vi "test - copy state with replace option.vi"(8 "error in (no error)":errorcluster, 11 "TestCase in":refnum<class "testcase-csmhelper.lvclass">) -> (0 "error out":errorcluster, 3 "TestCase out":refnum<class "testcase-csmhelper.lvclass">)   [LabVIEW 2017, in "testcase-csmhelper.lvclass"]
uses:
  testcase-csmhelper.lvclass
  <vilib>/addons/_JKI Toolkits/VI Tester/TestCase.llb/TestCase.lvclass
  src/user.lib/_NEVSTOP/Communicable State Machine(CSM)/Communicable State Machine.lvlib
  C:/Program Files (x86)/National Instruments/LabVIEW 2017/vi.lib/addons/_JKI Toolkits/VI Tester/TestCase.llb/TestCase.lvclass
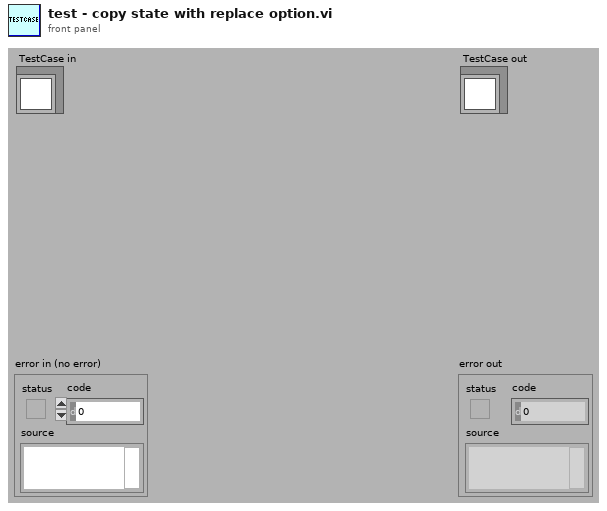
[diagram p1: front panel]
types:
  T1 = enum32{"Bad", "Idle", "Run top level", "Running"}
  T2 = cluster{"state":string, "error out":errorcluster, "Execution:State":enum32{"Bad", "Idle", "Run top level", "Running"}}[]
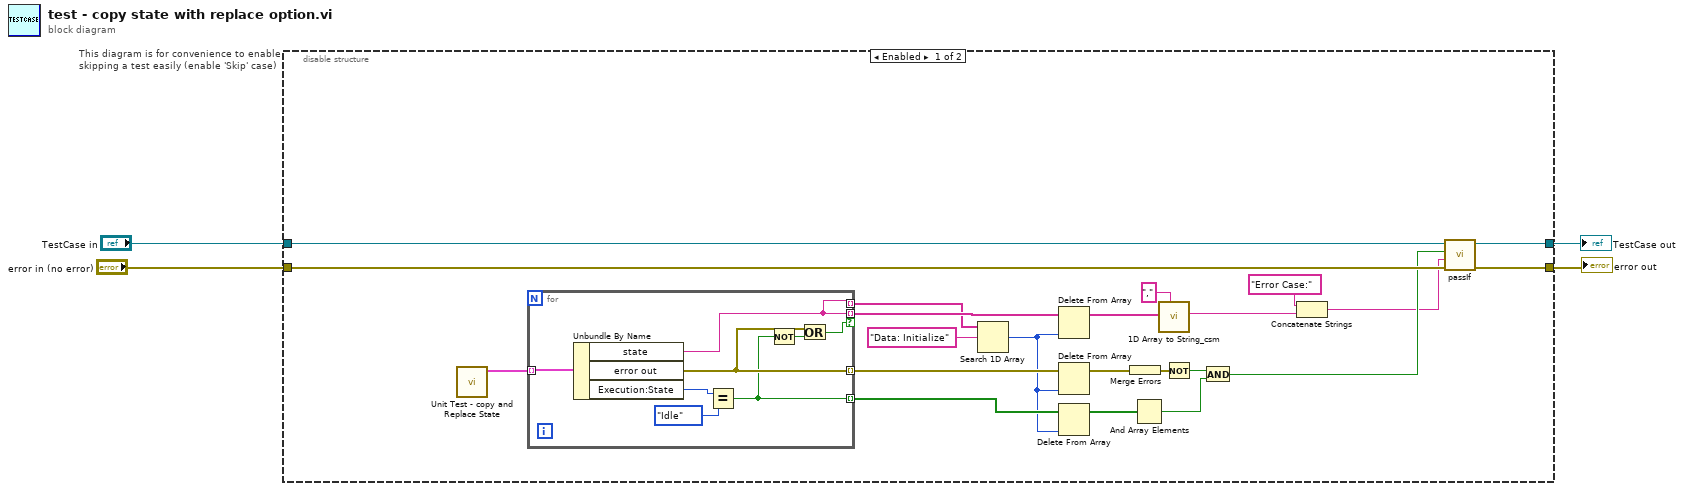
[diagram p0: block diagram]
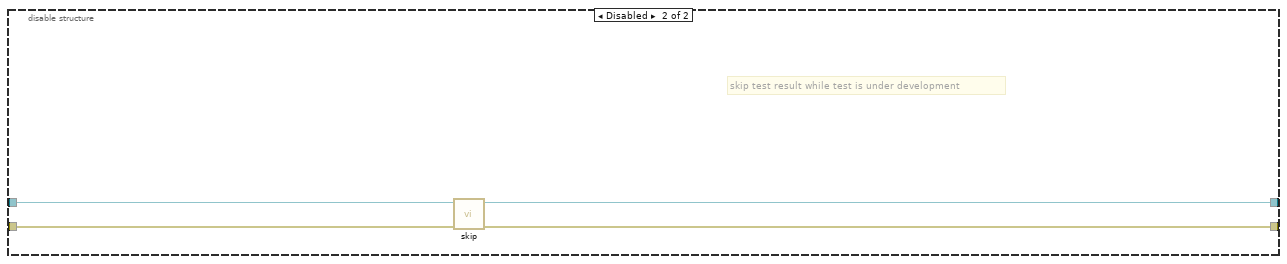
[diagram p2: hidden frame]
diagram:
  n1 = disable-structure "This diagram is for convenience to enable skipping a test easily (enable 'Skip' case)" shown="Enabled" {
    disable-tunnel: "TestCase in" -> [w22 w38]
    disable-tunnel: [w21 w36] -> w1
    disable-tunnel: [w19 w37] -> w3
    disable-tunnel: "error in (no error)" -> [w20 w35]
    frame Enabled {
      n2 = call "Unit Test - copy and Replace State.vi"() -> ("Array"=w26:T2)  [unwired: 11 in]
      n3 = for {
        tunnel: w26 -> [w34] mode=indexing
        tunnel: [w31] -> w10 mode=indexing
        tunnel: [w29] -> w12 mode=indexing
        tunnel: [w27] -> w8 mode=indexing if=w30
        tunnel: [w27] -> w5 mode=indexing
        n4 = Unbundle By Name(w34) -> ("state"=w27:string, "error out"=w31:errorcluster, "Execution:State"=w33:T1)
        n5 = Equal?(x=w33, y=T1."Idle") -> (x = y?=w29:bool)
        n6 = Not(x=w29) -> (.not. x?=w28:bool)
        n7 = Or(x=w31, y=w28) -> (x .or. y?=w30:bool)
      }
      n8 = Search 1D Array(1D array=w5, element="Data: Initialize") -> (index of element=w6:i32)  [unwired: 1 in]
      n9 = Delete From Array(array=w8, index=w6) -> (array with subset deleted=w7:string[])  [unwired: 1 in, 1 out]
      n10 = Delete From Array(array=w10, index=w6) -> (array with subset deleted=w9:errorcluster[])  [unwired: 1 in, 1 out]
      n11 = Delete From Array(array=w12, index=w6) -> (array with subset deleted=w11:bool[])  [unwired: 1 in, 1 out]
      n12 = Merge Errors(w9) -> (w25:errorcluster)
      n13 = And Array Elements(Boolean array=w11) -> (logical AND=w23:bool)
      n14 = call "1D Array to String_csm.vi"("delimiter (Tab)"=",", "Array of Strings"=w7) -> ("delimited string"=w17:string)  [unwired: 9 in]
      n15 = Not(x=w25) -> (.not. x?=w24:bool)
      n16 = And(x=w24, y=w23) -> (x .and. y?=w18:bool)
      n17 = Concatenate Strings("Error Case:" ("string"), w17) -> (w15:string)
      n18 = call-dynamic "passIf.vi"("error in (no error)"=w20, "message (\"\")"=w15, "pass"=w18, "TestCase in"=w22) -> ("error out"=w19:errorcluster, "TestCase out"=w21:refnum<class "testcase-csmhelper.lvclass">)  [unwired: 6 in]
    }
    frame Disabled {
      # "skip test result while test is under development"
      n19 = call <vilib>:"skip.vi"("error in (no error)"=w35, "TestCase in"=w38) -> ("error out"=w37:errorcluster, "TestCase out"=w36:refnum<class "testcase-csmhelper.lvclass">)  [unwired: 8 in]
    }
  }
  "error out" <- w3
  "TestCase out" <- w1
